vi "OF state.vi"(8 "errin":errorcluster, 11 "OF":string) -> (0 "error out":errorcluster, 2 "number string":string, 3 "number dbl":dbl)   [LabVIEW 2020]
doc: "Récupere l'état de l'OF"
uses:
  subVI/VarGLO/Global var.vi
  <vilib>/addons/database/Connection.llb/DB Tools Open Connec (String).vi
  <vilib>/addons/database/Connection.llb/Conn Execute.vi
  <vilib>/addons/database/Recordset.llb/Rec Fetch Recordset Data (R).vi
  <vilib>/addons/database/Recordset.llb/Rec Destroy - Connection.vi
  <vilib>/addons/database/NI_Database_API.lvlib
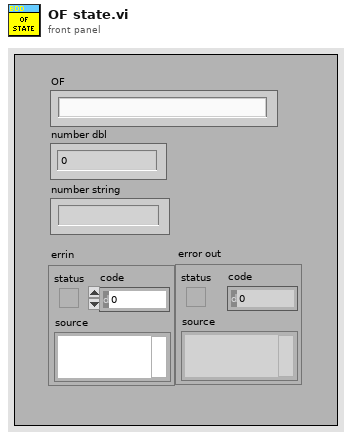
[diagram p1: front panel]
types:
  T1 = typedef "NI_Database_API.lvlib/Conn ObjectReference.ctl" = refnum<k1>
  T2 = typedef "NI_Database_API.lvlib/Rec ObjectReference.ctl" = refnum<k1>
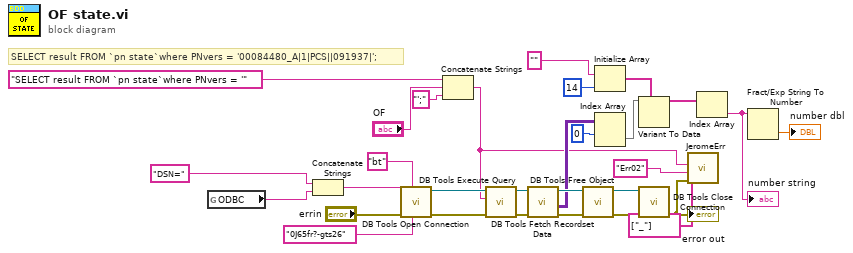
[diagram p0: block diagram]
diagram:
  # "SELECT result FROM `pn state`where PNvers = '00084480_A|1|PCS||091937|';"
  n1 = global read "Global var.vi" "ODBC"() -> (w1:string)
  n2 = Concatenate Strings("DSN=", w1) -> (w3:string)
  n3 = call-poly <vilib>:"DB Tools Open Connection.vi"("password"="0J65fr?-gts26", "userID"="bt", "error in (no error)"="errin", "connection information"=w3) -> ("error out"=w30:errorcluster, "connection reference"=w28:T1)  [unwired: 4 in]
  n4 = Concatenate Strings("SELECT result FROM `pn state`where PNvers = '" ("SQL query"), "OF", "';" ("chaîne")) -> (w6:string)
  n5 = call-poly <vilib>:"DB Tools Execute Query.vi"("error in (no error)"=w30, "SQL query"=w6, "connection reference"=w28) -> ("error out"=w24:errorcluster, "recordset reference"=w23:T2)  [unwired: 5 in]
  n6 = call-poly <vilib>:"DB Tools Fetch Recordset Data.vi"("error in (no error)"=w24, "recordset reference"=w23) -> ("error out"=w25:errorcluster, "recordset data"=w17:variant[][], "recordset reference out"=w22:T2)  [unwired: 3 in]
  n7 = call-poly <vilib>:"DB Tools Free Object.vi"("error in (no error)"=w25, "recordset reference"=w22) -> ("error out"=w29:errorcluster, "connection reference"=w27:T1)  [unwired: 8 in]
  n8 = Initialize Array("", 14 ("taille de la dimension")) -> (w13:string[])
  n9 = Index Array(array=w17, index (row)=0 ("indice (ligne)")) -> (element=w15:variant[])  [unwired: 1 in]
  n10 = Variant To Data ("Variant en donnée")(type=w13, Variant=w15) -> (data=w5:string[])  [unwired: 1 in, 1 out]
  n11 = call <vilib>:"DB Tools Close Connection.vi"("error in (no error)"=w29, "connection reference"=w27) -> ("error out"=w7:errorcluster)  [unwired: 5 in]
  "error out" <- w7
  n12 = call "JeromeErr.vi"("Errin"=w7, "CodeERR"="Err02", "RequetteSQL"=w6, "RetourSQL"=string[] ["_"]) -> ()  [unwired: 8 in]
  n13 = Index Array(array=w5) -> (element=w11:string)  [unwired: 1 in]
  "number string" <- w11
  n14 = Fract/Exp String To Number ("Chaîne Fract/Exp en nombre")(string=w11) -> (number=→"number dbl":dbl)  [unwired: 3 in, 1 out]
